vi "WSVCAP SHL FPGA LL Procedure I2C - Send Start or Stop Sequence.vi"(0 "Procedure Step":T1, 1 "Wait Ticks Remaining":u32, 5 "I2C Wait Ticks":u32, 11 "error in (no error)":errorcluster, 12 "Type (T:Start; F:Stop)":bool, 13 "Socket Mask":u64, 14 "UUT Set (0/1)":u8) -> (3 "Wait Ticks Remaining Out":u32, 4 "Procedure Step Out":T1, 8 "Finished":bool, 15 "error out":errorcluster)   [LabVIEW 2012]
uses:
  Type Defs/WSVCAP SHL Procedure Step Enum.ctl
  Type Defs/WSVCAP SHL I2C Write Line Enum.ctl
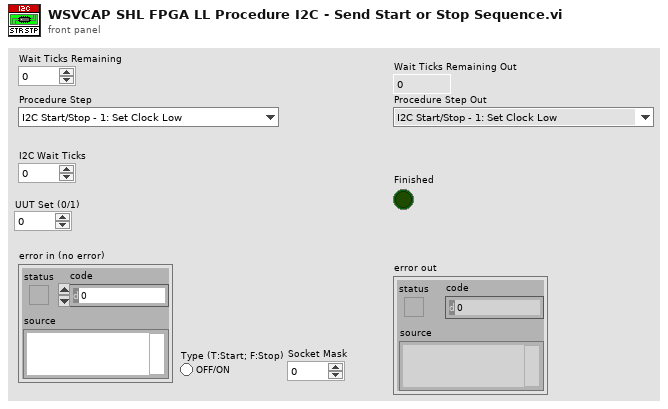
[diagram p1: front panel]
types:
  T1 = typedef "WSVCAP SHL Procedure Step Enum.ctl" = enum16{"I2C Start/Stop - 1: Set Clock Low", "I2C Start/Stop - 2: Wait", "I2C Start/Stop - 3: Set Data I", "I2C Start/Stop - 4: Wait", "I2C Start/Stop - 5: Set Clock High", "I2C Start/Stop - 6: Wait", "I2C Start/Stop - 7: Set Data II", "I2C Start/Stop - 8: Wait", "I2C Start/Stop - 9: Set Clock Low", "I2C Start/Stop - 10: Wait", "I2C Read ACK - 1: Set Clock High", "I2C Read ACK - 2: Wait", "I2C Read ACK - 3: Read ACK Bit", "I2C Read ACK - 4: Wait", "I2C Read ACK - 5: Set Clock Low", "I2C Read ACK - 6: Wait", "I2C Write ACK - 1: Write ACK Bit", "I2C Write ACK - 2: Wait", "I2C Write ACK - 3: Set Clock High", "I2C Write ACK - 4: Wait", "I2C Write ACK - 5: Set Clock Low", "I2C Write ACK - 6: Wait", "I2C Write ACK - 7: Set Data Low", "I2C Send Add - 1: Reset Bits Remaining", "I2C Send Add - 2: Set Data Bit", "I2C Send Add - 3: Wait", "I2C Send Add - 4: Set Clock High", "I2C Send Add - 5: Wait", "I2C Send Add - 6: Set Clock Low", "I2C Send Add - 7: Wait", "I2C Send Add - 8: Check Bits Remaining", "I2C Send Data - 1: Reset Bits Remaining", "I2C Send Data - 2: Load Write Bit from FIFO", "I2C Send Data - 3: Set Data Bit", "I2C Send Data - 4: Wait", "I2C Send Data - 5: Set Clock High", "I2C Send Data - 6: Wait", "I2C Send Data - 7: Set Clock Low", "I2C Send Data - 8: Wait", "I2C Send Data - 9: Check Bits Remaining", "I2C Receive Data - 1: Reset Bits Remaining", "I2C Receive Data - 2: Wait", "I2C Receive Data - 3: Set Clock High", "I2C Receive Data - 4: Wait", "I2C Receive Data - 5: Read Data Bit", "I2C Receive Data - 6: Wait", "I2C Receive Data - 7: Set Clock Low", "I2C Receive Data - 8: Wait", "I2C Receive Data - 9: Check Bits Remaining", "RFFE Send SSC - 1:Set Low", "RFFE Send SSC - 2:Wait", "RFFE Send SSC - 3:Set SDA High", "RFFE Send SSC - 4:Wait", "RFFE Send SSC - 5:Set SDA Low", "RFFE Send SSC - 6:Wait", "RFFE Send Data - 1:Set SCL High", "RFFE Send Data - 2:Wait", "RFFE Send Data - 3:Set SCL Low", "RFFE Send Data - 4:Wait", "RFFE Send Data - 5:Set SCL High (P)", "RFFE Send Data - 6:Wait", "RFFE Send Data - 7:Set SCL Low (P)", "RFFE Send Data - 8:Wait", "RFFE Send Data - 9:Set SCL High (BP)", "RFFE Send Data - 10:Wait", "RFFE Send Data - 11:Set SCL Low (BP)", "RFFE Send Data - 12:Wait", "RFFE Receive Data - 1:Set SCL High", "RFFE Receive Data - 2:Wait", "RFFE Receive Data - 3:Set SCL Low", "RFFE Receive Data - 4:Wait", "RFFE Receive Data - 5:Set SCL High (BP)", "RFFE Receive Data - 6:Wait", "RFFE Receive Data - 7:Set SCL Low (BP)", "RFFE Receive Data - 8:Wait", "RFFE Wait CMD Delay - 1:Wait", "RFFE Clear Lines - 1:Clear"}
  T2 = typedef "WSVCAP SHL I2C Write Line Enum.ctl" = enum16{"I2C SCL", "I2C SDA"}
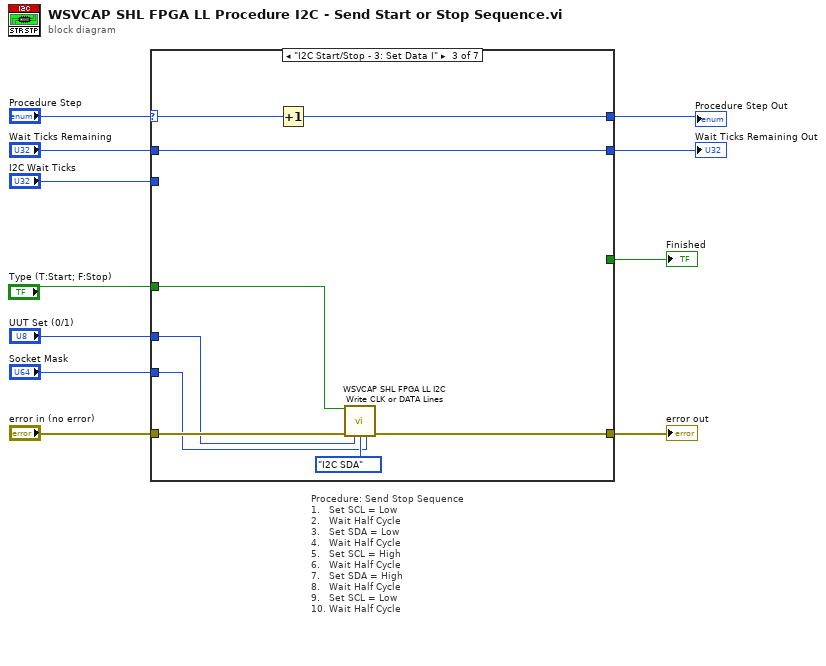
[diagram p0: block diagram]
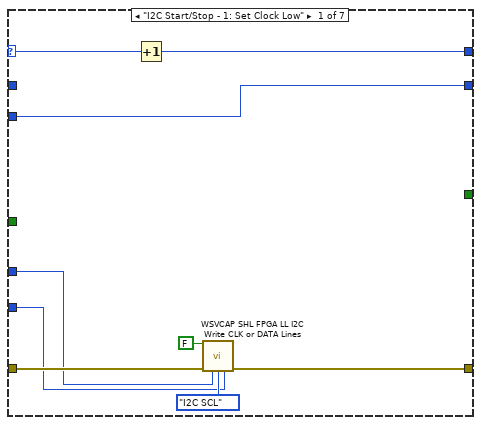
[diagram p2: hidden frame]
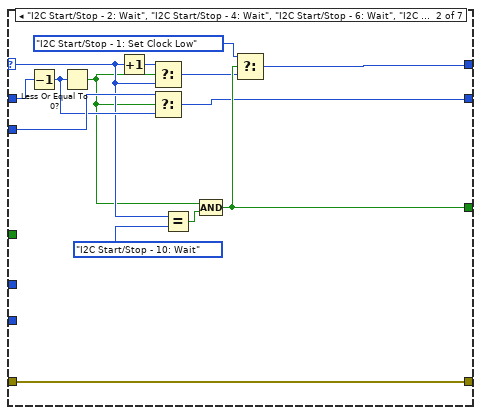
[diagram p3: hidden frame]
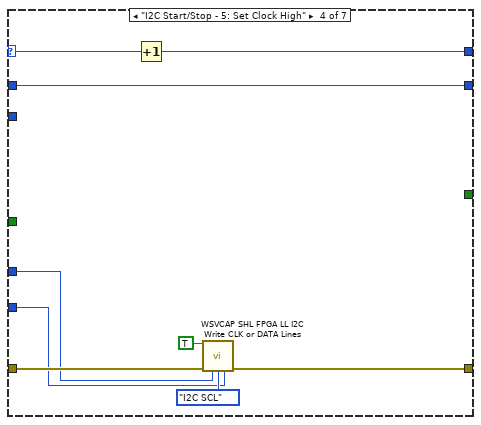
[diagram p4: hidden frame]
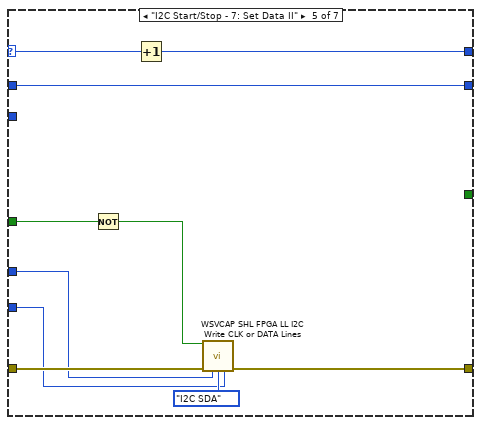
[diagram p5: hidden frame]
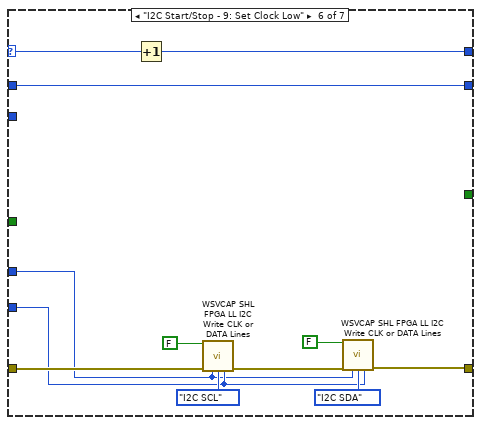
[diagram p6: hidden frame]
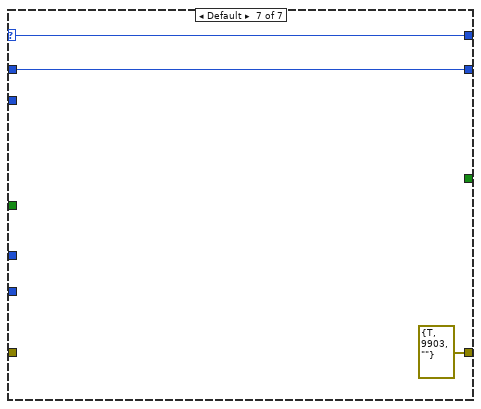
[diagram p7: hidden frame]
diagram:
  # "Procedure: Send Stop Sequence\n1.   Set SCL = Low\n2.   Wait Half Cycle\n3.   Set SDA = Low\n4.   Wait Half Cycle\n5.   Set SCL = High\n6.   Wait Half Cycle\n7.   Set SDA = High\n8.   Wait Half Cycle\n9.   Set SCL = Low\n10. Wait Half Cycle"
  n1 = case shown="\"I2C Start/Stop - 3: Set Data I\"" "Procedure Step" {
    selector: "Procedure Step" -> [w16 w29 w40 w48 w59 w71 w76]
    tunnel: [w18 w32 w41 w50 w60 w67 errorcluster {"status"=TRUE, "code"=9903, "source"=""} ("error out")] -> w10
    tunnel: "error in (no error)" -> [w19 w32 w42 w51 w61 w73 _]
    tunnel: "Wait Ticks Remaining" -> [_ w34 w36 w45 w54 w64 w75]
    tunnel: "I2C Wait Ticks" -> [w13 w31 _ _ _ _ _]
    tunnel: [_ w26 _ _ _ _ _] -> w9
    tunnel: "Socket Mask" -> [w15 _ w39 w47 w57 w66 _]
    tunnel: "Type (T:Start; F:Stop)" -> [_ _ w38 _ w56 _ _]
    tunnel: [w14 w22 w37 w46 w55 w65 w76] -> w3
    tunnel: [w13 w21 w36 w45 w54 w64 w75] -> w2
    tunnel: "UUT Set (0/1)" -> [w12 _ w35 w44 w53 w63 _]
    frame "I2C Start/Stop - 1: Set Clock Low" {
      n2 = Increment(x=w16) -> (x+1=w14:T1)
      n3 = call "WSVCAP SHL FPGA LL I2C Write CLK or DATA Lines.vi"("Bit In"=FALSE, "error in (no error)"=w19, "UUT Set (0/1)"=w12, "Line"=WSVCAP_SHL_I2C_Write_Line_Enum."I2C SCL", "Socket Mask"=w15) -> ("error out"=w18:errorcluster)  [unwired: 10 in]
    }
    frame "I2C Start/Stop - 2: Wait", "I2C Start/Stop - 4: Wait", "I2C Start/Stop - 6: Wait", "I2C Start/Stop - 8: Wait", "I2C Start/Stop - 10: Wait" {
      n4 = Decrement(x=w34) -> (x-1=w30:u32)
      n5 = Less Or Equal To 0?(x=w30) -> (x <= 0?=w28:bool)
      n6 = Increment(x=w29) -> (x+1=w33:T1)
      n7 = Select(t=w33, s=w28, f=w29) -> (s? t:f=w25:T1)
      n8 = Select(t=w31, s=w28, f=w30) -> (s? t:f=w21:u32)
      n9 = Equal?(x=w29, y=WSVCAP_SHL_Procedure_Step_Enum."I2C Start/Stop - 10: Wait" ("Procedure Step")) -> (x = y?=w27:bool)
      n10 = Compound Arithmetic op=AND(w28, w27) -> (w26:bool)
      n11 = Select(t=WSVCAP_SHL_Procedure_Step_Enum."I2C Start/Stop - 1: Set Clock Low" ("Procedure Step"), s=w26, f=w25) -> (s? t:f=w22:T1)
    }
    frame "I2C Start/Stop - 3: Set Data I" {
      n12 = Increment(x=w40) -> (x+1=w37:T1)
      n13 = call "WSVCAP SHL FPGA LL I2C Write CLK or DATA Lines.vi"("Bit In"=w38, "error in (no error)"=w42, "UUT Set (0/1)"=w35, "Line"=WSVCAP_SHL_I2C_Write_Line_Enum."I2C SDA", "Socket Mask"=w39) -> ("error out"=w41:errorcluster)  [unwired: 10 in]
    }
    frame "I2C Start/Stop - 5: Set Clock High" {
      n14 = Increment(x=w48) -> (x+1=w46:T1)
      n15 = call "WSVCAP SHL FPGA LL I2C Write CLK or DATA Lines.vi"("Bit In"=TRUE, "error in (no error)"=w51, "UUT Set (0/1)"=w44, "Line"=WSVCAP_SHL_I2C_Write_Line_Enum."I2C SCL", "Socket Mask"=w47) -> ("error out"=w50:errorcluster)  [unwired: 10 in]
    }
    frame "I2C Start/Stop - 7: Set Data II" {
      n16 = Not(x=w56) -> (.not. x?=w58:bool)
      n17 = Increment(x=w59) -> (x+1=w55:T1)
      n18 = call "WSVCAP SHL FPGA LL I2C Write CLK or DATA Lines.vi"("Bit In"=w58, "error in (no error)"=w61, "UUT Set (0/1)"=w53, "Line"=WSVCAP_SHL_I2C_Write_Line_Enum."I2C SDA", "Socket Mask"=w57) -> ("error out"=w60:errorcluster)  [unwired: 10 in]
    }
    frame "I2C Start/Stop - 9: Set Clock Low" {
      n19 = Increment(x=w71) -> (x+1=w65:T1)
      n20 = call "WSVCAP SHL FPGA LL I2C Write CLK or DATA Lines.vi"("Bit In"=FALSE, "error in (no error)"=w73, "UUT Set (0/1)"=w63, "Line"=WSVCAP_SHL_I2C_Write_Line_Enum."I2C SCL", "Socket Mask"=w66) -> ("error out"=w68:errorcluster)  [unwired: 10 in]
      n21 = call "WSVCAP SHL FPGA LL I2C Write CLK or DATA Lines.vi"("Bit In"=FALSE, "error in (no error)"=w68, "UUT Set (0/1)"=w63, "Line"=WSVCAP_SHL_I2C_Write_Line_Enum."I2C SDA", "Socket Mask"=w66) -> ("error out"=w67:errorcluster)  [unwired: 10 in]
    }
    frame Default {
    }
  }
  "error out" <- w10
  "Finished" <- w9
  "Wait Ticks Remaining Out" <- w2
  "Procedure Step Out" <- w3
